vi "configure processor core.vi"() -> (3 "Processor":i32)   [LabVIEW 2013]
uses:
  <vilib>/Utility/RT CPU pool selections.ctl
  <vilib>/NI_Real-Time Target Support.lvlib
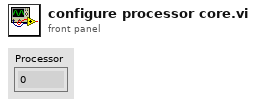
[diagram p1: front panel]
types:
  T1 = typedef "NI_Real-Time Target Support.lvlib/RT CPU pool selections.ctl" = enum16{"System & Timed Structures", "System", "Timed Structures", "Reserved"}
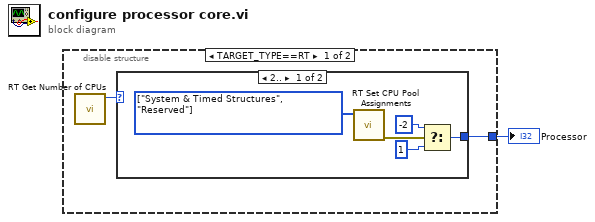
[diagram p0: block diagram]
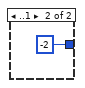
[diagram p2: hidden frame]
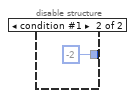
[diagram p3: hidden frame]
diagram:
  n1 = disable-structure shown="TARGET_TYPE==RT" {
    disable-tunnel: [w2 -2 ("Processor")] -> w1
    frame condition #0 (active) {
      n2 = call <vilib>:"RT Get Number of CPUs.vi"() -> ("# of CPUs"=w3:u32)  [unwired: 10 in, 1 out]
      n3 = case shown="2.." w3 {
        tunnel: [w6 -2 ("Processor")] -> w2
        frame 2.. {
          w8 = T1[] [enum."System & Timed Structures", enum."Reserved"] items=["System & Timed Structures", "System", "Timed Structures", "Reserved"] ("CPU pools")
          n4 = call <vilib>:"RT Set CPU Pool Assignments.vi"("CPU pools"=w8) -> ("error out"=w5:errorcluster)  [unwired: 7 in, 3 out]
          n5 = Select(t=-2, s=w5, f=1 ("Processor")) -> (s? t:f=w6:i32)
        }
        frame ..1 {
        }
      }
    }
    frame condition #1 {
    }
  }
  "Processor" <- w1
